vi "Remove JSON Tag.vi"(11 "Name":string) -> (2 "Tag":T1, 3 "Name (tag stripped)":string)   [LabVIEW 2019, in "JSONtext.lvlib"]
uses:
  JSONtext.lvlib
  Tag Type.ctl
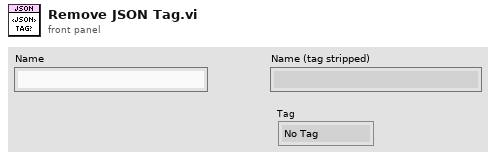
[diagram p1: front panel]
types:
  T1 = typedef "JSONtext.lvlib/Tag Type.ctl" = enum16{"No Tag", "<JSON>", "<JOBJ>"}
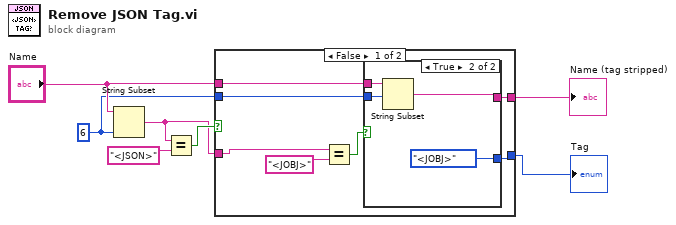
[diagram p0: block diagram]
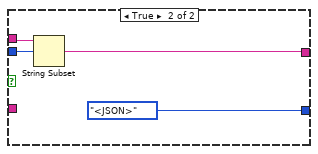
[diagram p3: hidden frame]
diagram:
  w3 = 6 ("length (rest)")
  n1 = String Subset(string="Name", length (rest)=w3) -> (substring=w2:string)  [unwired: 1 in]
  n2 = Equal?(x=w2, y="<JSON>") -> (x = y?=w7:bool)
  n3 = case shown="False" w7 {
    tunnel: [w11 w22] -> w5
    tunnel: "Name" -> [w12 w23]
    tunnel: w3 -> [w10 w21]
    tunnel: w2 -> [w13 _]
    tunnel: [w8 Tag_Type."<JSON>" ("Tag")] -> w1
    frame False {
      n4 = Equal?(x=w13, y="<JOBJ>") -> (x = y?=w9:bool)
      n5 = case shown="True" w9 {
        tunnel: w12 -> [w15 w19]
        tunnel: [w15 w18] -> w11
        tunnel: w10 -> [_ w17]
        tunnel: [_ Tag_Type."<JOBJ>" ("Tag")] -> w8
        frame False {
        }
        frame True {
          n6 = String Subset(string=w19, offset (0)=w17) -> (substring=w18:string)  [unwired: 1 in]
        }
      }
    }
    frame True {
      n7 = String Subset(string=w23, offset (0)=w21) -> (substring=w22:string)  [unwired: 1 in]
    }
  }
  "Tag" <- w1
  "Name (tag stripped)" <- w5
